vi "Drop Down VI Loader.vi"(7 "Software Config File Path":path) -> ()   [LabVIEW 2016]
uses:
  Drop Down VI Loader Type Defs/DDVL Drop Down Bar.ctl
  <vilib>/Utility/miscctls.llb/LVPointTypeDef.ctl
  <vilib>/Utility/miscctls.llb/LVRectTypeDef.ctl
panel:
  in  "Hide Exit Bar":bool
  in  "Hide Drop Bars":bool
  in  "Screen and Exit Bar":T1
  in  "Drop Down Control 1":T2
  in  "Drop Down Control 2":T2
  in  "Drop Down Control 3":T2
  in  "Drop Down Control 4":T2
  in  "Drop Down Control 5":T2
  in  "Drop Down Control 6":T2
  in  "Drop Down Control 7":T2
  in  "Drop Down Control 8":T2
  in  "Drop Down Control 9":T2
  in  "Drop Down Control 10":T2
  # "Device Panel"
  # "Focus / Alignment"
  # "Capture Manager"
  # "XY Control"
  # "Objective Img Align"
  # "DM Control"
  # "Interference Locator"
  # "Astig Align"
  # "Objective Lock"
  # "Some Text"
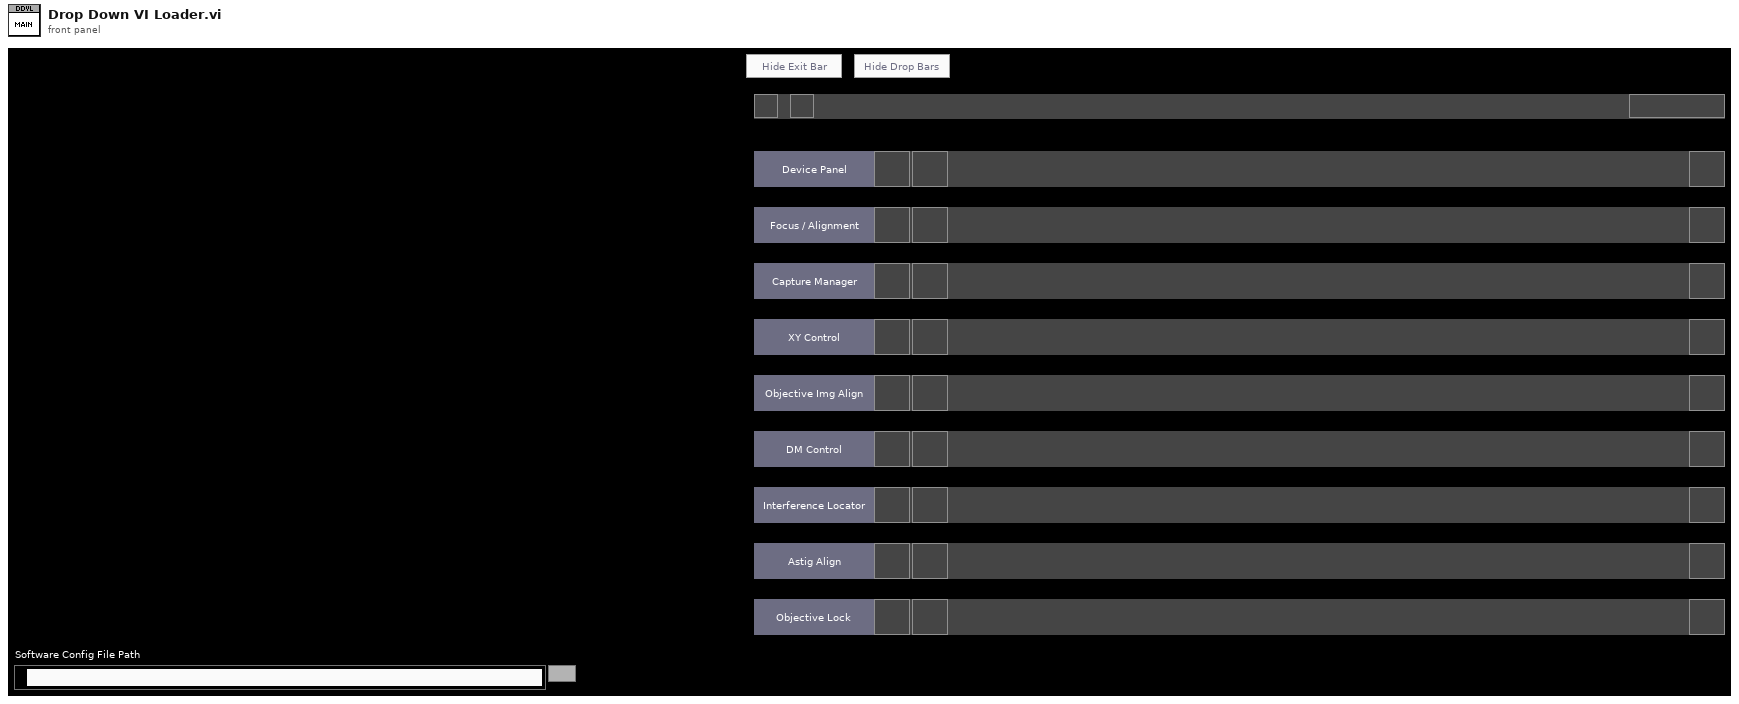
[diagram p1: front panel]
types:
  T1 = cluster{"Max Left":bool, "Max Right":bool, "Exit":bool, "Messages":string}
  T2 = typedef "DDVL Drop Down Bar.ctl" = cluster{"Right Width":bool, "Messages":string, "Abort VI":bool, "Close VI":bool}
  T3 = enum16{"Always On", "Always Off", "Off While Running"}
  T4 = typedef "LVPointTypeDef.ctl" = cluster{"Horizontal":i16, "Vertical":i16}
  T5 = enum32{"Invalid", "Standard", "Closed", "Hidden", "Minimized", "Maximized"}
  T6 = typedef "LVRectTypeDef.ctl" = cluster{"Left":i16, "Top":i16, "Right":i16, "Bottom":i16}
  T7 = enum8{"Enabled", "Disabled", "Disabled and Grayed Out"}
  T8 = cluster{"VI Path":path, "VI Refnum":refnum<vi>}[]
  T9 = typedef "lveventtype.ctl" = enum32{"Null", "Timeout", "Annotation Menu Selection", "Annotation Menu Selection?", "App Instance Close", "App Instance Close?", "Autoscale Range Change", "Bookmark Info Change", "Cell Edit", "Cell Edit?", "Cursor Grab", "Cursor Grab?", "Cursor Menu Selection", "Cursor Menu Selection?", "Cursor Move", "Cursor Release", "Data Change", "Direction Change", "Display State Change", "Drag Ended", "Drag Enter", "Drag Leave", "Drag Over", "Drag Source Update", "Drag Starting", "Drag Starting?", "Drop", "Exec State Change", "Key Down", "Key Down?", "Key Repeat", "Key Repeat?", "Key Up", "Listbox Double Click", "Menu Activation?", "Menu Selection (App)", "Menu Selection? (App)", "Menu Selection (User)", "Mouse Down", "Mouse Down?", "Mouse Enter", "Mouse Leave", "Mouse Move", "Mouse Up", "Mouse Wheel", "NI Security User Change (App)", "Pane Size", "Panel Close", "Panel Close?", "Panel Resize", "Plot Attribute Change", "Scale Range Change", "Shortcut Menu Activation?", "Shortcut Menu Selection (App)", "Shortcut Menu Selection? (App)", "Shortcut Menu Selection (User)", "Tree Double Click", "Tree Drag", "Tree Drag?", "Tree Drop", "Tree Drop?", "Tree Item Close", "Tree Item Close?", "Tree Item Open", "Tree Item Open?", "User Event", "Value Change"}
  T10 = typedef "LVAllMonitorsDisplayTypeDef.ctl" = cluster{"Bounds":cluster{"Left":i16, "Top":i16, "Right":i16, "Bottom":i16}, "Depth":i16}[]
  T11 = cluster{"Bounds":cluster{"Left":i16, "Top":i16, "Right":i16, "Bottom":i16}, "Depth":i16}
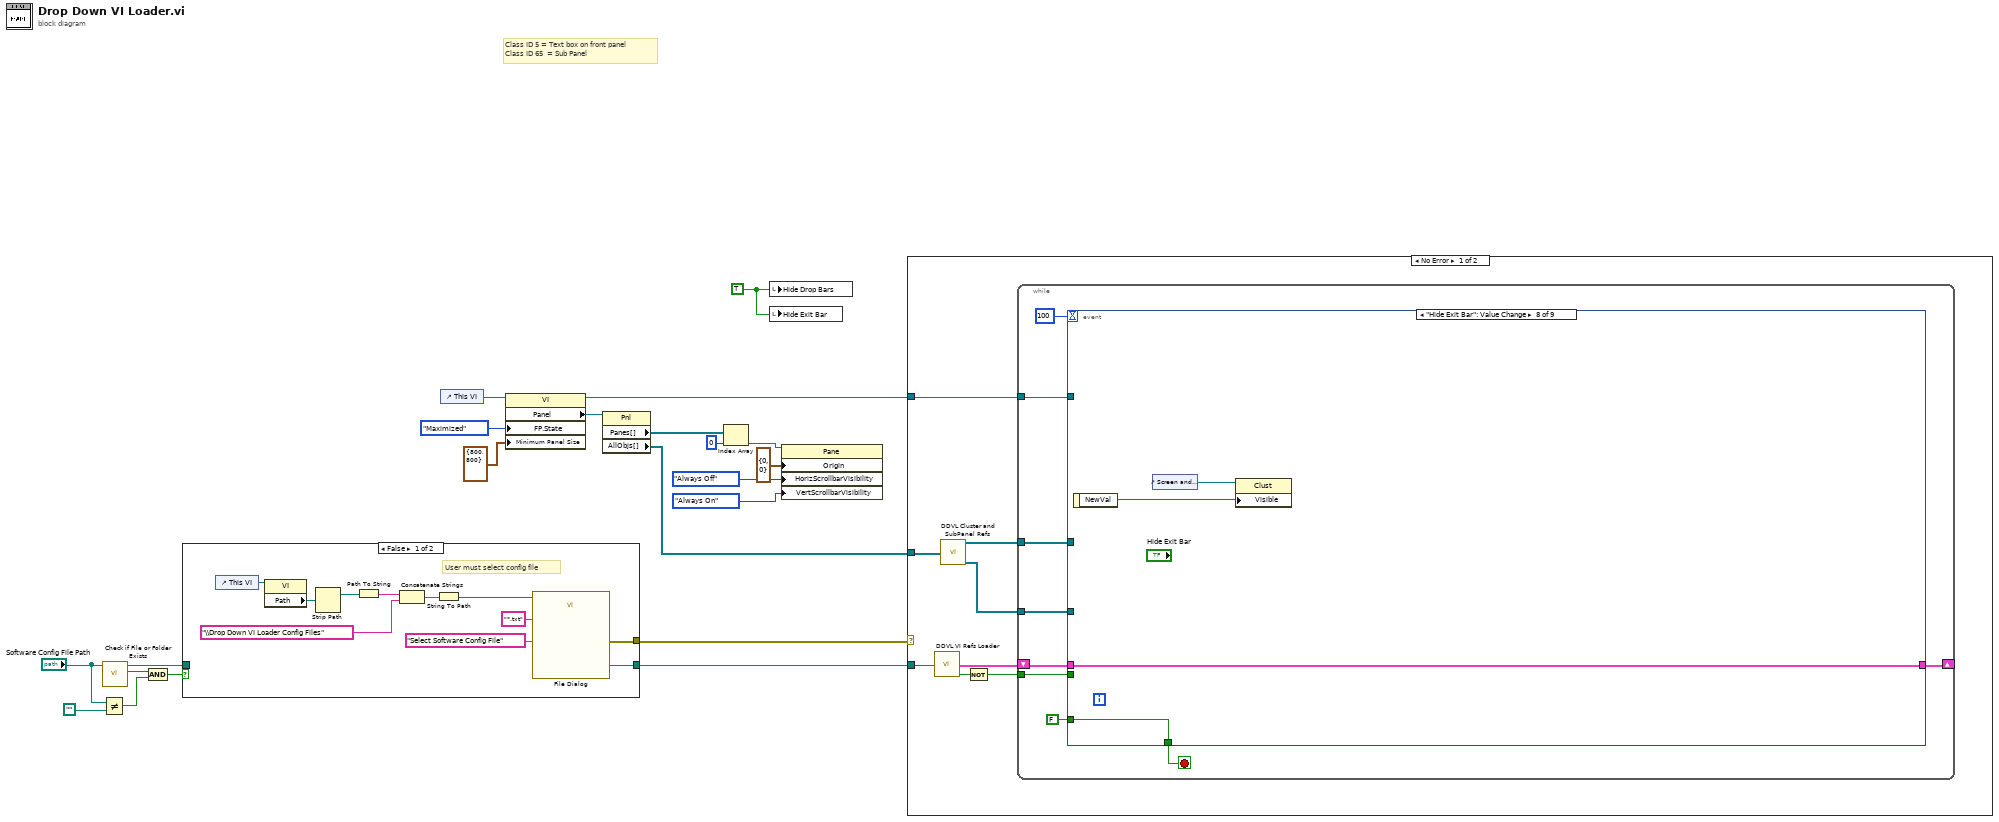
[diagram p0: block diagram]
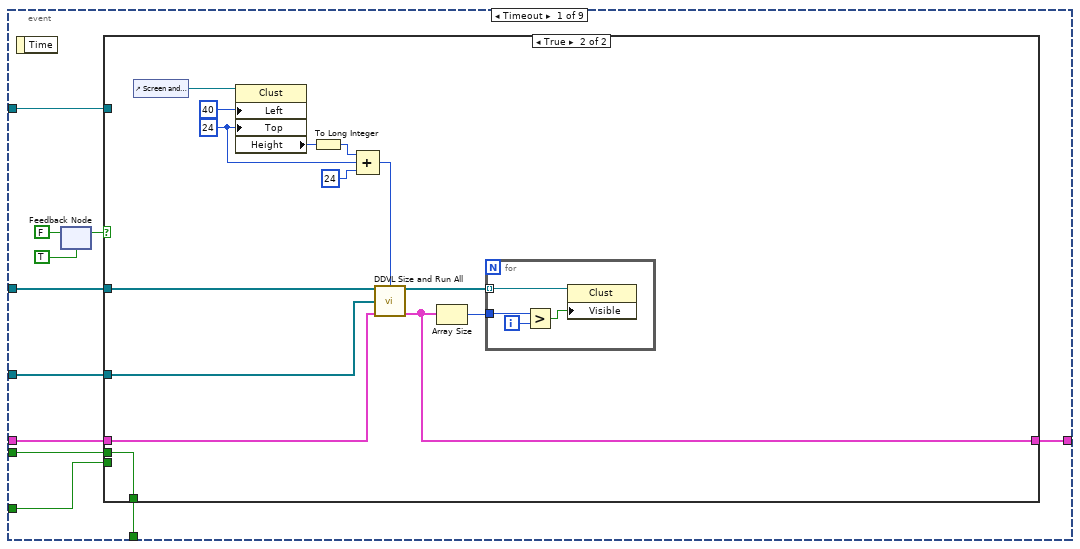
[diagram p2: hidden frame]
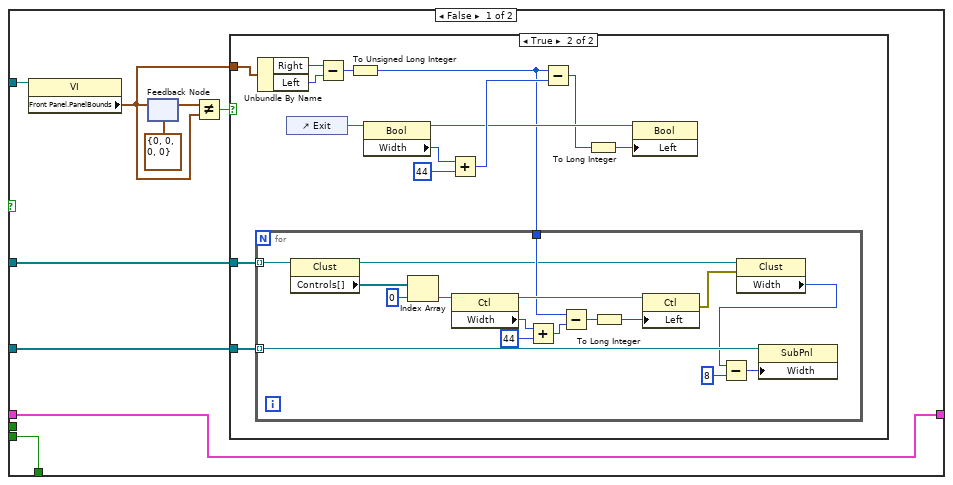
[diagram p3: hidden frame]
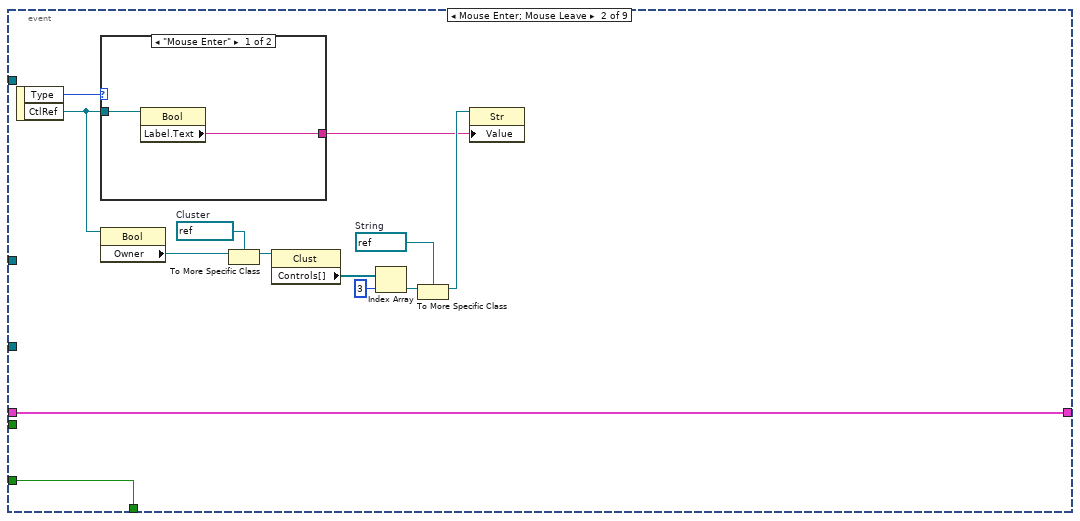
[diagram p5: hidden frame]
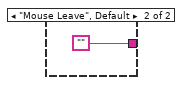
[diagram p6: hidden frame]
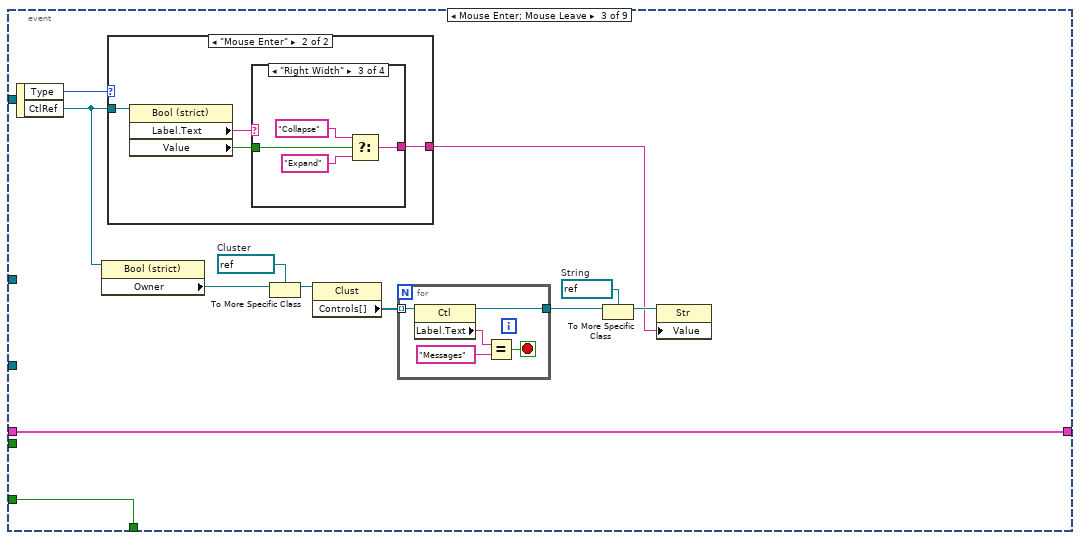
[diagram p7: hidden frame]
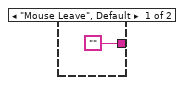
[diagram p8: hidden frame]
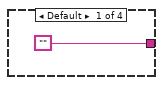
[diagram p9: hidden frame]
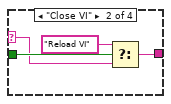
[diagram p10: hidden frame]
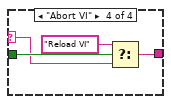
[diagram p11: hidden frame]
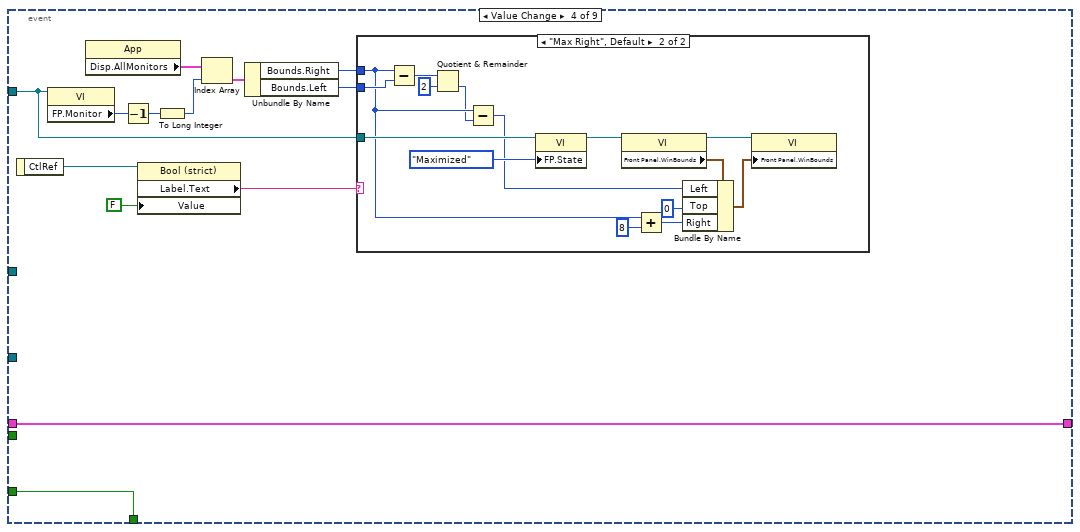
[diagram p12: hidden frame]
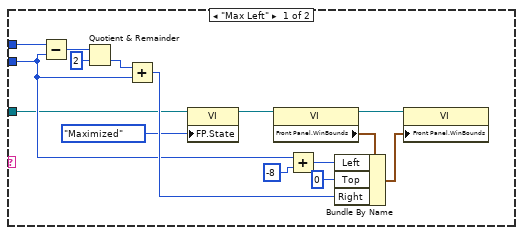
[diagram p13: hidden frame]
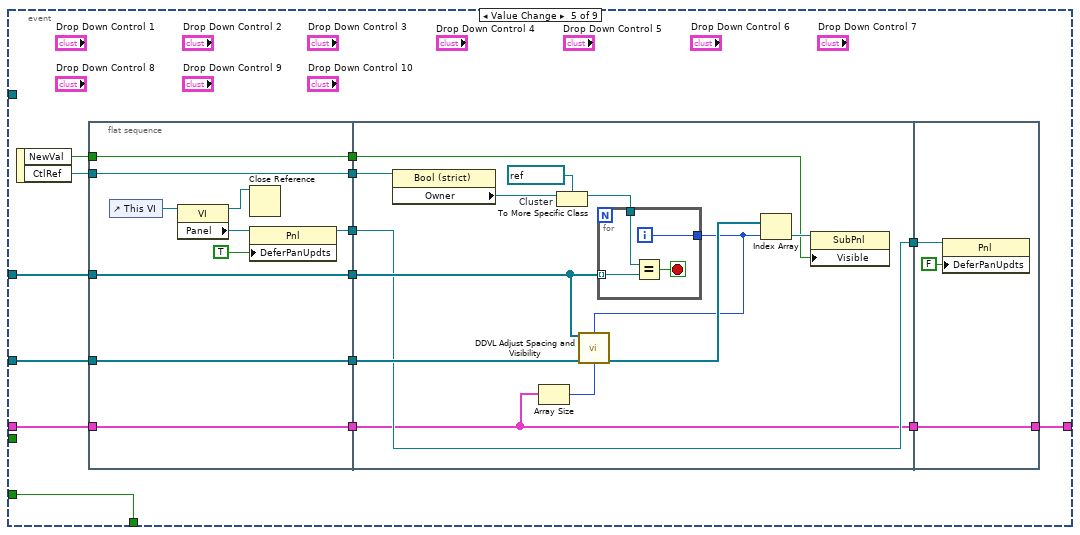
[diagram p14: hidden frame]
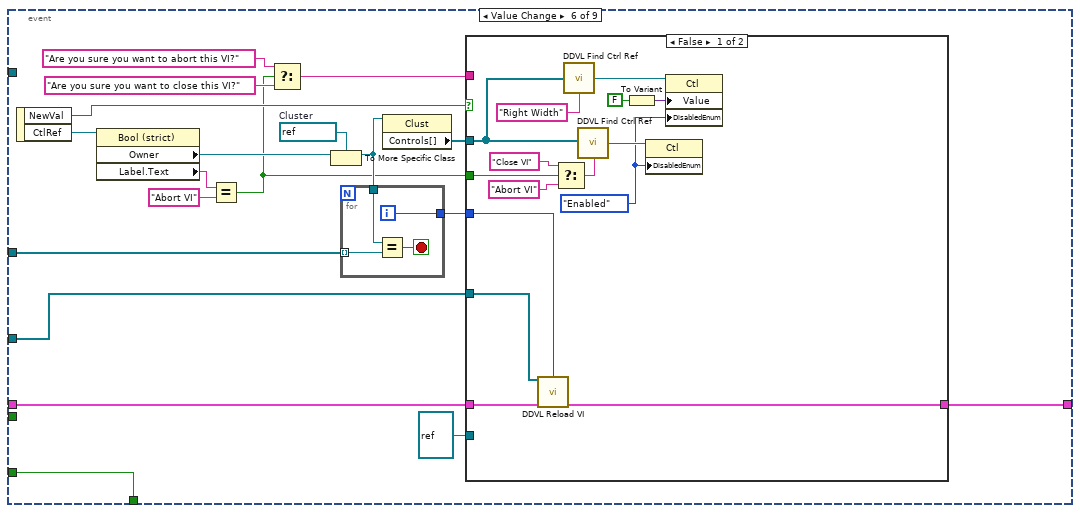
[diagram p15: hidden frame]
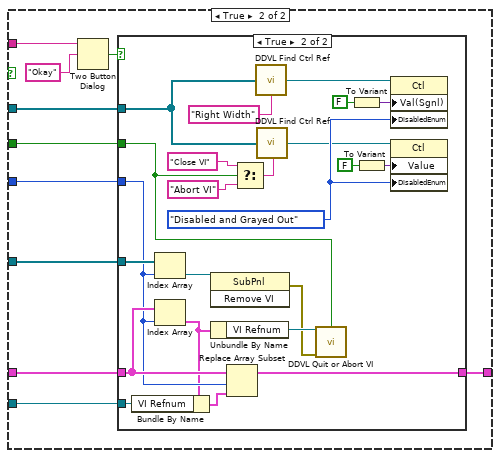
[diagram p16: hidden frame]
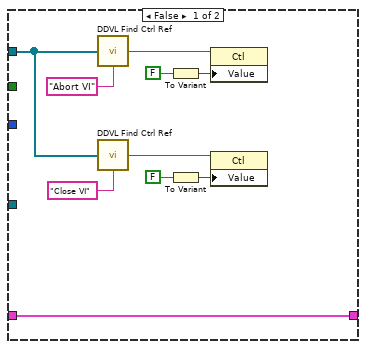
[diagram p17: hidden frame]
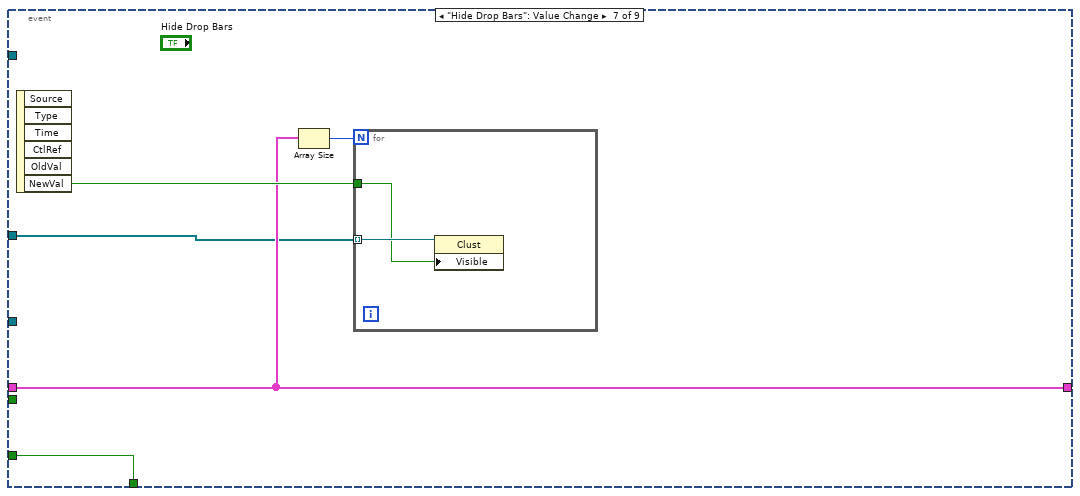
[diagram p18: hidden frame]
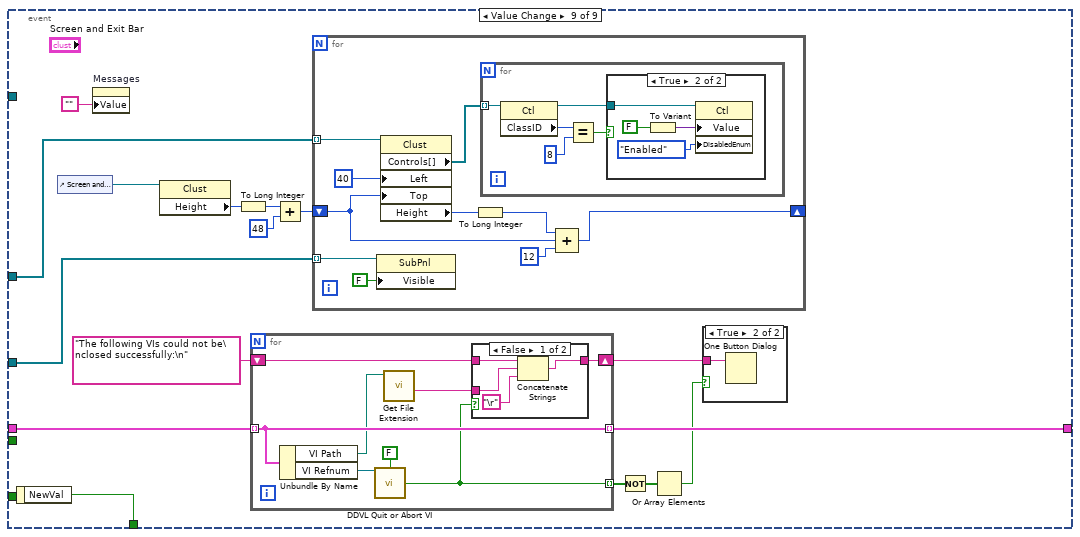
[diagram p19: hidden frame]
diagram:
  w1 = TRUE ("Hide Drop Bars")
  # "Class ID 5 = Text box on front panel\nClass ID 65  = Sub Panel"
  n1 = Not Equal?(x="Software Config File Path", y=path "") -> (x != y?=w8:bool)
  n2 = call <vilib>:"Check if File or Folder Exists.vi"("path"="Software Config File Path") -> ("file or folder exists?"=w7:bool, "dup path"=w5:path)  [unwired: 8 in, 1 out]
  n3 = And(x=w7, y=w8) -> (x .and. y?=w6:bool)
  n4 = case shown="False" w6 {
    tunnel: w5 -> [_ w34]
    tunnel: [w30 w34] -> w2
    tunnel: [w29 errorcluster {"status"=FALSE, "code"=0, "source"=""} ("error out")] -> w3
    frame False {
      # "User must select config file"
      n5 = control-ref of="This VI"() -> (w24:refnum<vi>)
      n6 = property class="VI"(reference=w24) -> ("Path"=w23:path)  [unwired: 1 in, 2 out]
      n7 = Strip Path(path=w23) -> (stripped path=w25:path)  [unwired: 1 out]
      n8 = Path To String(path=w25) -> (string=w26:string)
      n9 = Concatenate Strings(w26, "\\Drop Down VI Loader Config Files") -> (w28:string)
      n10 = String To Path(string=w28) -> (path=w22:path)
      n11 = call "File Dialog"("start path"=w22, "prompt"="Select Software Config File", "pattern (all files)"="*.txt") -> ("selected path"=w30:path, "error out"=w29:errorcluster)  [unwired: 9 in, 2 out]
    }
    frame True {
      # "Config File is specified - try and use it"
    }
  }
  n12 = control-ref of="This VI"() -> (w17:refnum<vi>)
  n13 = property class="VI"(reference=w17, "FP.State"=T5."Maximized" ("Front Panel Window:State"), "Minimum Panel Size"=T4 {"Horizontal"=800, "Vertical"=800} ("Front Panel Window:Minimum Size")) -> (reference out=w12:refnum<vi>, "Panel"=w11:refnum<vi>)  [unwired: 1 in, 1 out]
  n14 = property class="Pnl"(reference=w11) -> ("Panes[]"=w14:refnum<vi>[], "AllObjs[]"=w10:refnum<vi>[])  [unwired: 1 in, 2 out]
  n15 = Index Array(array=w14, index=0) -> (element=w20:refnum<vi>)
  n16 = local write "Hide Drop Bars"(w1) -> ()
  n17 = local write "Hide Exit Bar"(w1) -> ()
  n18 = property class="Pane"(reference=w20, "Origin"=T4 {"Horizontal"=0, "Vertical"=0}, "HorizScrollbarVisibility"=T3."Always Off" ("Vertical Scrollbar Visibility"), "VertScrollbarVisibility"=T3."Always On" ("Vertical Scrollbar Visibility")) -> ()  [unwired: 1 in, 2 out]
  n19 = case shown="No Error" w3 {
    tunnel: w12 -> [w42 _]
    tunnel: w10 -> [w40 _]
    tunnel: w2 -> [w37 _]
    frame No Error {
      n20 = call "DDVL VI Refs Loader.vi"("Config File Path"=w37) -> ("VI Path/Ref"=w39:T8, "VIs Loaded?"=w41:bool)  [unwired: 12 in, 1 out]
      n21 = call "DDVL Cluster and SubPanel Refs.vi"("All Objects Refs"=w40) -> ("Cluster Refs"=w36:refnum<vi>[], "Sub Panel Refs"=w35:refnum<vi>[])  [unwired: 13 in]
      n22 = Not(x=w41) -> (.not. x?=w38:bool)
      n23 = while {
        tunnel: w42 -> [w48]
        tunnel: w36 -> [w43]
        tunnel: w35 -> [w46]
        tunnel: w38 -> [w45]
        shift-right: [w44] -> _
        shift-left: w39 -> [w47]
        stop <- w51 stop-if-true
        n24 = event shown="[7] \"Hide Exit Bar\": Value Change" {
          selector: _ -> [_ _ _ _ _ _ _ _ _]
          dyn-events: _ -> [_ _ _ _ _ _ _ _ _]
          timeout: 100 -> [_ _ _ _ _ _ _ _ _]
          tunnel: [w58 w133 w147 w184 w229 w278 w345 w351 w367] -> w51
          tunnel: FALSE -> [w57 w133 w147 w184 w229 w278 w345 w351 _]
          tunnel: w48 -> [w62 _ _ w175 _ _ _ _ _]
          tunnel: w43 -> [w61 _ _ _ w227 w273 w341 _ w365]
          tunnel: w46 -> [w60 _ _ _ w228 w271 _ _ w364]
          tunnel: w47 -> [w59 w121 w148 w172 w224 w272 w342 w350 w358]
          tunnel: w45 -> [w56 _ _ _ _ _ _ _ _]
          tunnel: [w55 w121 w148 w172 w216 w269 w342 w350 w357] -> w44
          event Timeout {
            n25 = event-data() -> ()  [unwired: 1 in, 1 out]
            n26 = feedback #1(TRUE) -> (w52:bool)
            n27 = feedback-in #1(FALSE) -> ()
            n28 = case shown="True" w52 {
              tunnel: w62 -> [w71 _]
              tunnel: w61 -> [w66 w107]
              tunnel: w60 -> [w65 w114]
              tunnel: w59 -> [w63 w113]
              tunnel: [w64 w104] -> w58
              tunnel: w57 -> [w64 _]
              tunnel: w56 -> [_ w104]
              tunnel: [w63 w103] -> w55
              frame False {
                n29 = property class="VI"(reference=w71) -> ("Front Panel.PanelBounds"=w67:T6)  [unwired: 1 in, 2 out]
                n30 = feedback-in #2(w67) -> ()
                n31 = feedback #2(T6 {"Left"=0, "Top"=0, "Right"=0, "Bottom"=0} ("Front Panel.PanelBounds")) -> (w70:T6)
                n32 = Not Equal?(x=w70, y=w67) -> (x != y?=w68:bool)
                n33 = case shown="True" w68 {
                  tunnel: w67 -> [_ w85]
                  tunnel: w66 -> [_ w75]
                  tunnel: w65 -> [_ w72]
                  frame False {
                  }
                  frame True {
                    n34 = Unbundle By Name(w85) -> ("Right"=w77:i16, "Left"=w78:i16)
                    n35 = control-ref of="Exit"() -> (w83:refnum<vi>)
                    n36 = Subtract(x=w77, y=w78) -> (x-y=w76:i16)
                    n37 = To Unsigned Long Integer(number=w76) -> (unsigned 32bit integer=w73:u32)
                    n38 = for {
                      tunnel: w75 -> [w102] mode=indexing
                      tunnel: w73 -> [w93]
                      tunnel: w72 -> [w91] mode=indexing
                      n39 = property class="Clust"(reference=w102) -> (reference out=w90:refnum<vi>, "Controls[]"=w101:refnum<vi>[])  [unwired: 1 in, 1 out]
                      n40 = Index Array(array=w101, index=0) -> (element=w97:refnum<vi>)
                      n41 = property class="Ctl"(reference=w97) -> (reference out=w96:refnum<vi>, "Width"=w98:u32)  [unwired: 1 in, 1 out]
                      n42 = Add(x=w98, y=u32 44) -> (x+y=w95:u32)
                      n43 = Subtract(x=w93, y=w95) -> (x-y=w94:u32)
                      n44 = To Long Integer(number=w94) -> (32bit integer=w99:i32)
                      n45 = property class="Ctl"(reference=w96, "Left"=w99) -> (error out=w89:errorcluster)  [unwired: 1 in, 1 out]
                      n46 = property class="Clust"(reference=w90, error in=w89) -> ("Width"=w88:u32)  [unwired: 2 out]
                      n47 = Subtract(x=w88, y=u32 8) -> (x-y=w87:u32)
                      n48 = property class="SubPnl"(reference=w91, "Width"=w87) -> ()  [unwired: 1 in, 2 out]
                    }
                    n49 = property class="Bool"(reference=w83) -> (reference out=w81:refnum<vi>, "Width"=w84:u32)  [unwired: 1 in, 1 out]
                    n50 = Add(x=w84, y=u32 44) -> (x+y=w82:u32)
                    n51 = Subtract(x=w73, y=w82) -> (x-y=w79:u32)
                    n52 = To Long Integer(number=w79) -> (32bit integer=w80:i32)
                    n53 = property class="Bool"(reference=w81, "Left"=w80) -> ()  [unwired: 1 in, 2 out]
                  }
                }
              }
              frame True {
                w111 = 24 ("Position:Top")
                n54 = control-ref of="Screen and Exit Bar"() -> (w116:refnum<vi>)
                n55 = property class="Clust"(reference=w116, "Left"=40 ("Position:Left"), "Top"=w111) -> ("Height"=w112:u32)  [unwired: 1 in, 2 out]
                n56 = To Long Integer(number=w112) -> (32bit integer=w110:i32)
                n57 = Compound Arithmetic op=ADD(w110, w111, 24 ("value")) -> (w108:i32)
                n58 = call "DDVL Size and Run All.vi"("Cluster Refs"=w107, "Initial Top Position"=w108, "Subpanel Refs"=w114, "VI Path/Ref"=w113) -> ("Cluster Refs Dup"=w106:refnum<vi>[], "VI Path/Ref Out"=w103:T8)  [unwired: 10 in]
                n59 = Array Size(array=w103) -> (size(s)=w105:i32)
                n60 = for {
                  tunnel: w106 -> [w120] mode=indexing
                  tunnel: w105 -> [w117]
                  i -> [w119]
                  n61 = Greater?(x=w117, y=w119) -> (0:w118:bool)
                  n62 = property class="Clust"(reference=w120, "Visible"=w118) -> ()  [unwired: 1 in, 2 out]
                }
              }
            }
          }
          event "Screen and Exit Bar.Exit", "Screen and Exit Bar.Max Right", "Screen and Exit Bar.Max Left": Mouse Enter; "Screen and Exit Bar.Exit", "Screen and Exit Bar.Max Right", "Screen and Exit Bar.Max Left": Mouse Leave {
            w124 = refnum<vi> refnum  # String
            w129 = refnum<vi> refnum  # Cluster
            n63 = event-data() -> ("Type"=w132:T9, "CtlRef"=w131:refnum<vi>)  [unwired: 1 in]
            n64 = case shown="\"Mouse Enter\"" w132 {
              tunnel: w131 -> [w135 _]
              tunnel: [w134 ""] -> w122
              frame "Mouse Enter" {
                n65 = property class="Bool"(reference=w135) -> ("Label.Text"=w134:string)  [unwired: 1 in, 2 out]
              }
              frame "Mouse Leave", Default {
              }
            }
            n66 = property class="Bool"(reference=w131) -> ("Owner"=w130:refnum<vi>)  [unwired: 1 in, 2 out]
            n67 = To More Specific Class(target class=w129, reference=w130) -> (specific class reference=w128:refnum<vi>)  [unwired: 1 in, 1 out]
            n68 = property class="Clust"(reference=w128) -> ("Controls[]"=w127:refnum<vi>[])  [unwired: 1 in, 2 out]
            n69 = Index Array(array=w127, index=3) -> (element=w125:refnum<vi>)
            n70 = To More Specific Class(target class=w124, reference=w125) -> (specific class reference=w123:refnum<vi>)  [unwired: 1 in, 1 out]
            n71 = property class="Str"(reference=w123, "Value"=w122) -> ()  [unwired: 1 in, 2 out]
          }
          event Mouse Enter; Mouse Leave {
            w139 = refnum<vi> refnum  # String
            w144 = refnum<vi> refnum  # Cluster
            n72 = event-data() -> ("Type"=w146:T9, "CtlRef"=w145:refnum<vi>)  [unwired: 1 in]
            n73 = property class="Bool (strict)"(reference=w145) -> ("Owner"=w142:refnum<vi>)  [unwired: 1 in, 2 out]
            n74 = case shown="\"Mouse Enter\"" w146 {
              tunnel: w145 -> [_ w158]
              tunnel: ["" w155] -> w137
              frame "Mouse Leave", Default {
              }
              frame "Mouse Enter" {
                n75 = property class="Bool (strict)"(reference=w158) -> ("Label.Text"=w157:string, "Value"=w156:bool)  [unwired: 1 in, 2 out]
                n76 = case shown="\"Right Width\"" w157 {
                  selector: w157 -> [_ w162 _ w169]
                  tunnel: w156 -> [_ w163 w167 w170]
                  tunnel: ["" w160 w164 w168] -> w155
                  frame Default {
                  }
                  frame "Close VI" {
                    n77 = Select(t="Reload VI", s=w163, f=w162) -> (s? t:f=w160:string)
                  }
                  frame "Right Width" {
                    n78 = Select(t="Collapse", s=w167, f="Expand") -> (s? t:f=w164:string)
                  }
                  frame "Abort VI" {
                    n79 = Select(t="Reload VI", s=w170, f=w169) -> (s? t:f=w168:string)
                  }
                }
              }
            }
            n80 = To More Specific Class(target class=w144, reference=w142) -> (specific class reference=w143:refnum<vi>)  [unwired: 1 in, 1 out]
            n81 = property class="Clust"(reference=w143) -> ("Controls[]"=w141:refnum<vi>[])  [unwired: 1 in, 2 out]
            n82 = for {
              tunnel: w141 -> [w153] mode=indexing
              tunnel: [w149] -> w140
              stop <- w150 stop-if-true
              n83 = property class="Ctl"(reference=w153) -> (reference out=w149:refnum<vi>, "Label.Text"=w152:string)  [unwired: 1 in, 1 out]
              n84 = Equal?(x=w152, y="Messages") -> (x = y?=w150:bool)
            }
            n85 = To More Specific Class(target class=w139, reference=w140) -> (specific class reference=w138:refnum<vi>)  [unwired: 1 in, 1 out]
            n86 = property class="Str"(reference=w138, "Value"=w137) -> ()  [unwired: 1 in, 2 out]
          }
          event "Screen and Exit Bar.Max Right", "Screen and Exit Bar.Max Left": Value Change {
            n87 = event-data() -> ("CtlRef"=w183:refnum<vi>)  [unwired: 1 in]
            n88 = property class="VI"(reference=w175) -> ("FP.Monitor"=w182:u16)  [unwired: 1 in, 2 out]
            n89 = property class="App"() -> ("Disp.AllMonitors"=w181:T10)  [unwired: 2 in, 2 out]
            n90 = Decrement(x=w182) -> (x-1=w180:u16)
            n91 = property class="Bool (strict)"(reference=w183, "Value"=FALSE) -> ("Label.Text"=w174:string)  [unwired: 1 in, 2 out]
            n92 = To Long Integer(number=w180) -> (32bit integer=w179:i32)
            n93 = Index Array(array=w181, index=w179) -> (element=w178:T11)
            n94 = Unbundle By Name(w178) -> ("Bounds.Right"=w177:i16, "Bounds.Left"=w176:i16)
            n95 = case shown="\"Max Right\", Default" w174 {
              tunnel: w177 -> [w199 w202]
              tunnel: w176 -> [w187 w206]
              tunnel: w175 -> [w185 w205]
              frame "Max Left" {
                n96 = Subtract(x=w199, y=w187) -> (x-y=w194:i16)
                n97 = Quotient & Remainder(x=w194, y=i16 2) -> (floor(x/y)=w192:i16)  [unwired: 1 out]
                n98 = Add(x=w192, y=w187) -> (x+y=w191:i16)
                n99 = property class="VI"(reference=w185, "FP.State"=T5."Maximized" ("Front Panel Window:State")) -> (reference out=w189:refnum<vi>)  [unwired: 1 in, 1 out]
                n100 = property class="VI"(reference=w189) -> (reference out=w198:refnum<vi>, "Front Panel.WinBounds"=w196:T6)  [unwired: 1 in, 1 out]
                n101 = Add(x=w187, y=i16 -8 ("Left")) -> (x+y=w186:i16)
                n102 = Bundle By Name(cluster=w196, "Left"=w186, "Top"=i16 0, "Right"=w191) -> (w197:T6)
                n103 = property class="VI"(reference=w198, "Front Panel.WinBounds"=w197) -> ()  [unwired: 1 in, 2 out]
              }
              frame "Max Right", Default {
                n104 = Subtract(x=w202, y=w206) -> (x-y=w211:i16)
                n105 = Quotient & Remainder(x=w211, y=i16 2) -> (floor(x/y)=w201:i16)  [unwired: 1 out]
                n106 = Subtract(x=w202, y=w201) -> (x-y=w200:i16)
                n107 = property class="VI"(reference=w205, "FP.State"=T5."Maximized" ("Front Panel Window:State")) -> (reference out=w208:refnum<vi>)  [unwired: 1 in, 1 out]
                n108 = property class="VI"(reference=w208) -> (reference out=w214:refnum<vi>, "Front Panel.WinBounds"=w212:T6)  [unwired: 1 in, 1 out]
                n109 = Add(x=w202, y=i16 8 ("Left")) -> (x+y=w203:i16)
                n110 = Bundle By Name(cluster=w212, "Left"=w200, "Top"=i16 0, "Right"=w203) -> (w213:T6)
                n111 = property class="VI"(reference=w214, "Front Panel.WinBounds"=w213) -> ()  [unwired: 1 in, 2 out]
              }
            }
          }
          event Value Change {
            n112 = event-data() -> ("NewVal"=w225:bool, "CtlRef"=w226:refnum<vi>)  [unwired: 1 in]
            n113 = flat-sequence {
              tunnel: w224 -> [w235]
              tunnel: w225 -> [w236]
              tunnel: w226 -> [w237]
              tunnel: w227 -> [w238]
              tunnel: w228 -> [w239]
              tunnel: [w239] -> w223
              tunnel: [w238] -> w222
              tunnel: [w237] -> w221
              tunnel: [w236] -> w220
              tunnel: [w235] -> w219
              tunnel: [w230] -> w217
              tunnel: w223 -> [w250]
              tunnel: w222 -> [w249]
              tunnel: w221 -> [w248]
              tunnel: w220 -> [w244]
              tunnel: w219 -> [w240]
              tunnel: [w241] -> w218
              tunnel: w217 -> [w241]
              tunnel: [w240] -> w215
              tunnel: w218 -> [w259]
              tunnel: [w257] -> w216
              tunnel: w215 -> [w257]
              frame #0 {
                n114 = control-ref of="This VI"() -> (w232:refnum<vi>)
                n115 = property class="VI"(reference=w232) -> (reference out=w231:refnum<vi>, "Panel"=w233:refnum<vi>)  [unwired: 1 in, 1 out]
                n116 = Close Reference(reference=w231) -> ()  [unwired: 1 in, 1 out]
                n117 = property class="Pnl"(reference=w233, "DeferPanUpdts"=TRUE ("Defer Panel Updates")) -> (reference out=w230:refnum<vi>)  [unwired: 1 in, 1 out]
              }
              frame #1 {
                w246 = refnum<vi> refnum  # Cluster
                n118 = property class="Bool (strict)"(reference=w248) -> ("Owner"=w247:refnum<vi>)  [unwired: 1 in, 2 out]
                n119 = Array Size(array=w240) -> (size(s)=w242:i32)
                n120 = To More Specific Class(target class=w246, reference=w247) -> (specific class reference=w245:refnum<vi>)  [unwired: 1 in, 1 out]
                n121 = for {
                  tunnel: w249 -> [w256] mode=indexing
                  tunnel: w245 -> [w255]
                  tunnel: [w253] -> w243
                  i -> [w253]
                  stop <- w254 stop-if-true
                  n122 = Equal?(x=w255, y=w256) -> (x = y?=w254:bool)
                }
                n123 = call "DDVL Adjust Spacing and Visibility.vi"("Cluster Ref Array"=w249, "Position Index"=w243, "Sub Panel Ref Array"=w250, "Num of VIs"=w242) -> ("Sub Panel Ref Array Dup"=w252:refnum<vi>[])  [unwired: 11 in]
                n124 = Index Array(array=w252, index=w243) -> (element=w251:refnum<vi>)
                n125 = property class="SubPnl"(reference=w251, "Visible"=w244) -> ()  [unwired: 1 in, 2 out]
              }
              frame #2 {
                n126 = property class="Pnl"(reference=w259, "DeferPanUpdts"=FALSE ("Defer Panel Updates")) -> ()  [unwired: 1 in, 2 out]
              }
            }
          }
          event Value Change {
            w276 = refnum<vi> refnum  # Cluster
            n127 = event-data() -> ("NewVal"=w270:bool, "CtlRef"=w275:refnum<vi>)  [unwired: 1 in]
            n128 = property class="Bool (strict)"(reference=w275) -> ("Owner"=w277:refnum<vi>, "Label.Text"=w267:string)  [unwired: 1 in, 2 out]
            n129 = Equal?(x=w267, y="Abort VI" ("message")) -> (x = y?=w260:bool)
            n130 = Select(t="Are you sure you want to abort this VI?" ("message"), s=w260, f="Are you sure you want to close this VI?" ("message")) -> (s? t:f=w263:string)
            n131 = To More Specific Class(target class=w276, reference=w277) -> (specific class reference=w262:refnum<vi>)  [unwired: 1 in, 1 out]
            n132 = for {
              tunnel: w273 -> [w340] mode=indexing
              tunnel: w262 -> [w339]
              tunnel: [w337] -> w274
              i -> [w337]
              stop <- w338 stop-if-true
              n133 = Equal?(x=w339, y=w340) -> (x = y?=w338:bool)
            }
            n134 = property class="Clust"(reference=w262) -> ("Controls[]"=w261:refnum<vi>[])  [unwired: 1 in, 2 out]
            n135 = case shown="False" w270 {
              tunnel: w274 -> [w290 w301]
              tunnel: w272 -> [w292 w300]
              tunnel: w271 -> [w293 w299]
              tunnel: w261 -> [w280 w295]
              tunnel: [w291 w298] -> w269
              tunnel: refnum<vi> refnum ("VI Refnum") -> [_ w297]
              tunnel: w263 -> [_ w296]
              tunnel: w260 -> [w286 w294]
              frame False {
                w279 = T7."Enabled" ("Disabled")
                n136 = call "DDVL Reload VI.vi"("Sub Panel Refs"=w293, "Index"=w290, "Path/Ref Array In"=w292) -> ("Updated Path/Ref Array"=w291:T8)  [unwired: 12 in]
                n137 = Select(t="Close VI" ("message"), s=w286, f="Abort VI" ("message")) -> (s? t:f=w287:string)
                n138 = call "DDVL Find Ctrl Ref.vi"("Control Array"=w280, "Control Label"="Right Width") -> ("Control Ref"=w283:refnum<vi>)  [unwired: 12 in, 1 out]
                n139 = call "DDVL Find Ctrl Ref.vi"("Control Array"=w280, "Control Label"=w287) -> ("Control Ref"=w285:refnum<vi>)  [unwired: 12 in, 1 out]
                n140 = To Variant(anything=FALSE) -> (Variant=w281:variant)
                n141 = property class="Ctl"(reference=w285, "DisabledEnum"=w279) -> ()  [unwired: 1 in, 2 out]
                n142 = property class="Ctl"(reference=w283, "Value"=w281, "DisabledEnum"=w279) -> ()  [unwired: 1 in, 2 out]
              }
              frame True {
                n143 = Two Button Dialog(message=w296, 2:"Okay" ("T button name (\"OK\")")) -> (T button?=w302:bool)  [unwired: 1 in]
                n144 = case shown="True" w302 {
                  tunnel: w301 -> [_ w331]
                  tunnel: w299 -> [_ w336]
                  tunnel: w300 -> [w313 w332]
                  tunnel: [w313 w329] -> w298
                  tunnel: w297 -> [_ w328]
                  tunnel: w295 -> [w307 w319]
                  tunnel: w294 -> [_ w321]
                  frame False {
                    n145 = call "DDVL Find Ctrl Ref.vi"("Control Array"=w307, "Control Label"="Abort VI") -> ("Control Ref"=w308:refnum<vi>)  [unwired: 12 in, 1 out]
                    n146 = call "DDVL Find Ctrl Ref.vi"("Control Array"=w307, "Control Label"="Close VI") -> ("Control Ref"=w306:refnum<vi>)  [unwired: 12 in, 1 out]
                    n147 = To Variant(anything=FALSE) -> (Variant=w311:variant)
                    n148 = To Variant(anything=FALSE) -> (Variant=w310:variant)
                    n149 = property class="Ctl"(reference=w308, "Value"=w311) -> ()  [unwired: 1 in, 2 out]
                    n150 = property class="Ctl"(reference=w306, "Value"=w310) -> ()  [unwired: 1 in, 2 out]
                  }
                  frame True {
                    w317 = T7."Disabled and Grayed Out" ("Disabled")
                    n151 = Index Array(array=w336, index=w331) -> (element=w335:refnum<vi>)
                    n152 = Index Array(array=w332, index=w331) -> (element=w327:cluster{"VI Path":path, "VI Refnum":refnum<vi>})
                    n153 = Bundle By Name(cluster=w327, "VI Refnum"=w328) -> (w330:cluster{"VI Path":path, "VI Refnum":refnum<vi>})
                    n154 = invoke class="SubPnl" method="Remove VI"(reference=w335) -> (error out=w322:errorcluster)  [unwired: 2 in, 2 out]
                    n155 = Unbundle By Name(w327) -> ("VI Refnum"=w323:refnum<vi>)
                    n156 = Replace Array Subset(array=w332, new element=w330, index=w331) -> (w329:T8)
                    n157 = Select(t="Close VI" ("message"), s=w321, f="Abort VI" ("message")) -> (s? t:f=w324:string)
                    n158 = call "DDVL Find Ctrl Ref.vi"("Control Array"=w319, "Control Label"="Right Width") -> ("Control Ref"=w318:refnum<vi>)  [unwired: 12 in, 1 out]
                    n159 = call "DDVL Find Ctrl Ref.vi"("Control Array"=w319, "Control Label"=w324) -> ("Control Ref"=w314:refnum<vi>)  [unwired: 12 in, 1 out]
                    n160 = call "DDVL Quit or Abort VI.vi"("VI Ref"=w323, "Abort VI?"=w321, "Error In"=w322) -> ()  [unwired: 12 in, 1 out]
                    n161 = To Variant(anything=FALSE) -> (Variant=w315:variant)
                    n162 = To Variant(anything=FALSE) -> (Variant=w334:variant)
                    n163 = property class="Ctl"(reference=w318, "Val(Sgnl)"=w315, "DisabledEnum"=w317) -> ()  [unwired: 1 in, 2 out]
                    n164 = property class="Ctl"(reference=w314, "Value"=w334, "DisabledEnum"=w317) -> ()  [unwired: 1 in, 2 out]
                  }
                }
              }
            }
          }
          event "Hide Drop Bars": Value Change {
            n165 = event-data() -> ("NewVal"=w344:bool)  [unwired: 1 in, 5 out]
            n166 = Array Size(array=w342) -> (size(s)=w343:i32)
            n167 = for {
              N: w343 -> [_]
              tunnel: w341 -> [w347] mode=indexing
              tunnel: w344 -> [w346]
              n168 = property class="Clust"(reference=w347, "Visible"=w346) -> ()  [unwired: 1 in, 2 out]
            }
          }
          event "Hide Exit Bar": Value Change {
            n169 = event-data() -> ("NewVal"=w348:bool)  [unwired: 1 in]
            n170 = control-ref of="Screen and Exit Bar"() -> (w349:refnum<vi>)
            n171 = property class="Clust"(reference=w349, "Visible"=w348) -> ()  [unwired: 1 in, 2 out]
          }
          event "Screen and Exit Bar.Exit": Value Change {
            n172 = event-data() -> ("NewVal"=w367:bool)  [unwired: 1 in]
            n173 = control-ref of="Screen and Exit Bar"() -> (w361:refnum<vi>)
            n174 = property on="Messages" class="Str"("Value"="") -> ()  [unwired: 2 in, 2 out]
            n175 = property class="Clust"(reference=w361) -> ("Height"=w360:u32)  [unwired: 1 in, 2 out]
            n176 = To Long Integer(number=w360) -> (32bit integer=w362:i32)
            n177 = for {
              tunnel: w358 -> [w376] mode=indexing
              tunnel: [w376] -> w357 mode=indexing
              shift-right: [w370] -> w352
              shift-left: "The following VIs could not be\nclosed successfully:\n" -> [w371]
              tunnel: [w369] -> w355 mode=indexing
              n178 = Unbundle By Name(w376) -> ("VI Path"=w373:path, "VI Refnum"=w375:refnum<vi>)
              n179 = call "DDVL Quit or Abort VI.vi"("VI Ref"=w375, "Abort VI?"=FALSE) -> ("Close Command Successful?"=w369:bool)  [unwired: 13 in]
              n180 = call <vilib>:"Get File Extension.vi"("file"=w373) -> ("filename without extension"=w372:string)  [unwired: 6 in, 4 out]
              n181 = case shown="False" w369 {
                tunnel: w372 -> [w379 _]
                tunnel: w371 -> [w378 w381]
                tunnel: [w377 w381] -> w370
                frame False {
                  n182 = Concatenate Strings(w378, w379, "\r") -> (w377:string)
                }
                frame True {
                }
              }
            }
            n183 = Add(x=w362, y=48) -> (x+y=w359:i32)
            n184 = for {
              tunnel: w365 -> [w390] mode=indexing
              shift-right: [w389] -> _
              shift-left: w359 -> [w385]
              tunnel: w364 -> [w382] mode=indexing
              n185 = property class="SubPnl"(reference=w382, "Visible"=FALSE) -> ()  [unwired: 1 in, 2 out]
              n186 = property class="Clust"(reference=w390, "Left"=40 ("Position:Left"), "Top"=w385) -> ("Controls[]"=w384:refnum<vi>[], "Height"=w387:u32)  [unwired: 1 in, 2 out]
              n187 = To Long Integer(number=w387) -> (32bit integer=w386:i32)
              n188 = for {
                tunnel: w384 -> [w396] mode=indexing
                n189 = property class="Ctl"(reference=w396) -> (reference out=w392:refnum<vi>, "ClassID"=w395:u32)  [unwired: 1 in, 1 out]
                n190 = Equal?(x=w395, y=u32 8) -> (x = y?=w393:bool)
                n191 = case shown="True" w393 {
                  tunnel: w392 -> [_ w398]
                  frame False {
                  }
                  frame True {
                    n192 = To Variant(anything=FALSE) -> (Variant=w399:variant)
                    n193 = property class="Ctl"(reference=w398, "Value"=w399, "DisabledEnum"=T7."Enabled" ("Disabled")) -> ()  [unwired: 1 in, 2 out]
                  }
                }
              }
              n194 = Compound Arithmetic op=ADD(w386, w385, 12 ("value")) -> (w389:i32)
            }
            n195 = Not(x=w355) -> (.not. x?=w354:bool[])
            n196 = Or Array Elements(Boolean array=w354) -> (logical OR=w353:bool)
            n197 = case shown="True" w353 {
              tunnel: w352 -> [_ w368]
              frame False {
              }
              frame True {
                n198 = One Button Dialog(message=w368) -> ()  [unwired: 1 in, 1 out]
              }
            }
          }
        }
      }
    }
    frame Error {
    }
  }
